vi "DeviceOn.vi"(8 "error in (no error)":errorcluster, 11 "ChromaPowerSupply in":refnum<class "ChromaPowerSupply.lvclass">) -> (0 "error out":errorcluster, 3 "ChromaPowerSupply out":refnum<class "ChromaPowerSupply.lvclass">)   [LabVIEW 2018, in "AcPwrPlugins.lvlib" / "ChromaPowerSupply.lvclass"]
doc: "This VI enables the instruments output to either generate or recieving a signal."
uses:
  ChromaPowerSupply.lvclass
  AcPwrBaseClass/AcPwrBase.lvclass
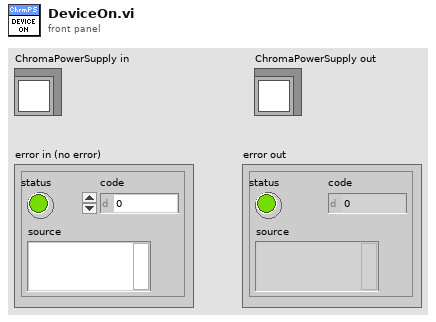
[diagram p1: front panel]
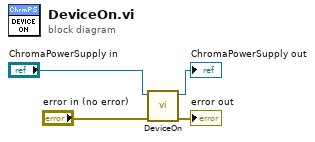
[diagram p0: block diagram]
diagram:
  n1 = call-parent "DeviceOn.vi"("error in (no error)"="error in (no error)", "AcPwrBase in"="ChromaPowerSupply in") -> ("error out"=→"error out":errorcluster, "AcPwrBase out"=→"ChromaPowerSupply out":refnum<class "ChromaPowerSupply.lvclass">)  [unwired: 8 in]
